vi "Configure Trigger Source.vi"(8 "error in (no error)":errorcluster, 9 "Trigger Source (0: Bus)":i32(ring) items=["Bus", "External", "Immediate", "Pin 1", "Pin 2", "Pin 3"], 10 "Channel (1)":string="1", 11 "VISA resource name":refnum<visa-resource-name>) -> (0 "error out":errorcluster, 3 "VISA resource name out":refnum<visa-resource-name>)   [LabVIEW 2020, in "Keysight E36300 Series.lvlib"]
doc: "Configures the trigger source for the output trigger system."
uses:
  Keysight E36300 Series.lvlib
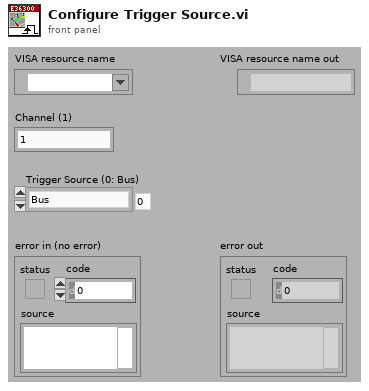
[diagram p1: front panel]
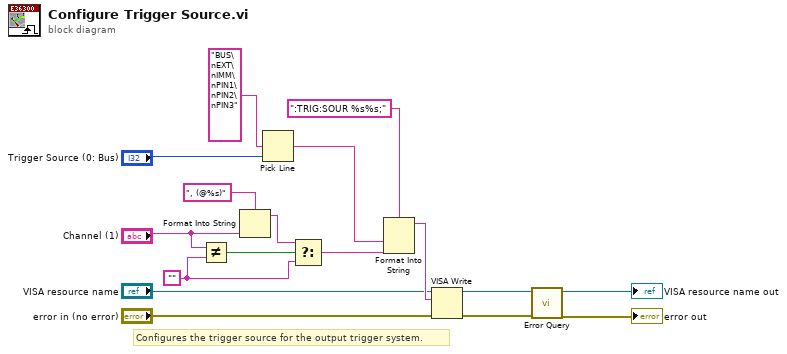
[diagram p0: block diagram]
diagram:
  w1 = ""
  # "Configures the trigger source for the output trigger system."
  n1 = Not Equal?(x="Channel (1)", y=w1) -> (x != y?=w4:bool)
  n2 = Format Into String(format string=", (@%s)", "Channel (1)") -> (resulting string=w5:string)  [unwired: 2 in, 1 out]
  n3 = Pick Line(multi-line string="BUS\nEXT\nIMM\nPIN1\nPIN2\nPIN3", line index="Trigger Source (0: Bus)") -> (output string=w15:string)  [unwired: 1 in]
  n4 = Select(t=w5, s=w4, f=w1) -> (s? t:f=w2:string)
  n5 = Format Into String(format string=":TRIG:SOUR %s%s;", w15, w2) -> (resulting string=w14:string)  [unwired: 2 in, 1 out]
  n6 = VISA Write(VISA resource name="VISA resource name", write buffer=w14, error in (no error)="error in (no error)") -> (VISA resource name out=w11:refnum<visa-resource-name>, error out=w10:errorcluster)  [unwired: 1 out]
  n7 = call "Error Query.vi"("error in (no error)"=w10, "VISA resource name"=w11) -> ("error out"=→"error out":errorcluster, "VISA resource name out"=→"VISA resource name out":refnum<visa-resource-name>)  [unwired: 6 in, 2 out]
